vi "Determine Bounds.vi"(8 "Lower Limit":dbl=0.05, 9 "Upper Limit":dbl=0.3, 11 "Input":dbl) -> (2 "Output":dbl)   [LabVIEW 2011]
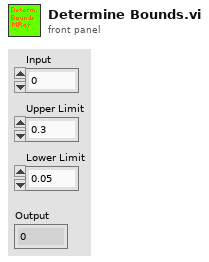
[diagram p1: front panel]
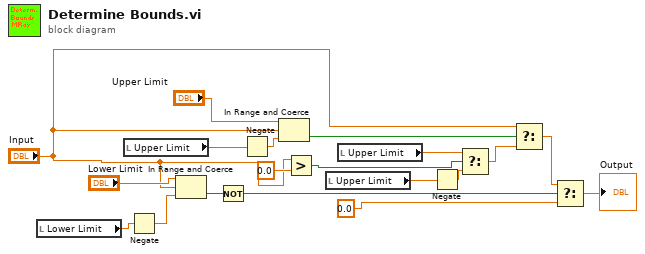
[diagram p0: block diagram]
diagram:
  n1 = local read "Lower Limit"() -> (w2:dbl)
  n2 = local read "Upper Limit"() -> (w14:dbl)
  n3 = Negate(x=w2) -> (-x=w1:dbl)
  n4 = In Range and Coerce(upper limit="Lower Limit", x="Input", lower limit=w1) -> (In Range?=w17:bool)  [unwired: 1 out]
  n5 = Not(x=w17) -> (.not. x?=w18:bool)
  n6 = Negate(x=w14) -> (-x=w13:dbl)
  n7 = In Range and Coerce(upper limit="Upper Limit", x="Input", lower limit=w13) -> (In Range?=w12:bool)  [unwired: 1 out]
  n8 = Greater?(x="Input", y=0.0) -> (0:w9:bool)
  n9 = local read "Upper Limit"() -> (w7:dbl)
  n10 = local read "Upper Limit"() -> (w8:dbl)
  n11 = Negate(x=w7) -> (-x=w6:dbl)
  n12 = Select(t=w8, s=w9, f=w6) -> (s? t:f=w5:dbl)
  n13 = Select(t="Input", s=w12, f=w5) -> (s? t:f=w10:dbl)
  n14 = Select(t=w10, s=w18, f=0.0) -> (s? t:f=→"Output":dbl)
